vi "Dio3232.vi"(7 "DIO3232_Action":T2, 8 "error in (no error)":errorcluster, 11 "I/Oin":T1 {"Port" items=["input_port0", "input_port1", "input_port2", "input_port3", "output_port0", "output_port1", "output_port2", "output_port3"]; "Point" max=31}) -> (0 "error out":errorcluster, 3 "I/O out":T1 {"Port" items=["input_port0", "input_port1", "input_port2", "input_port3", "output_port0", "output_port1", "output_port2", "output_port3"]})   [LabVIEW 2015]
uses:
  Dio3232_controls.ctl
panel:
  # "input_port0  ÂI¦ìinput0~7\ninput_port1  ÂI¦ìinput8~15\ninput_port2  ÂI¦ìinput16~23\ninput_port3  ÂI¦ìinput24~31"
  # "output_port0  ÂI¦ìoutput0~7\noutput_port1  ÂI¦ìoutput8~15\noutput_port2  ÂI¦ìoutput16~23\noutput_port3  ÂI¦ìoutput24~31"
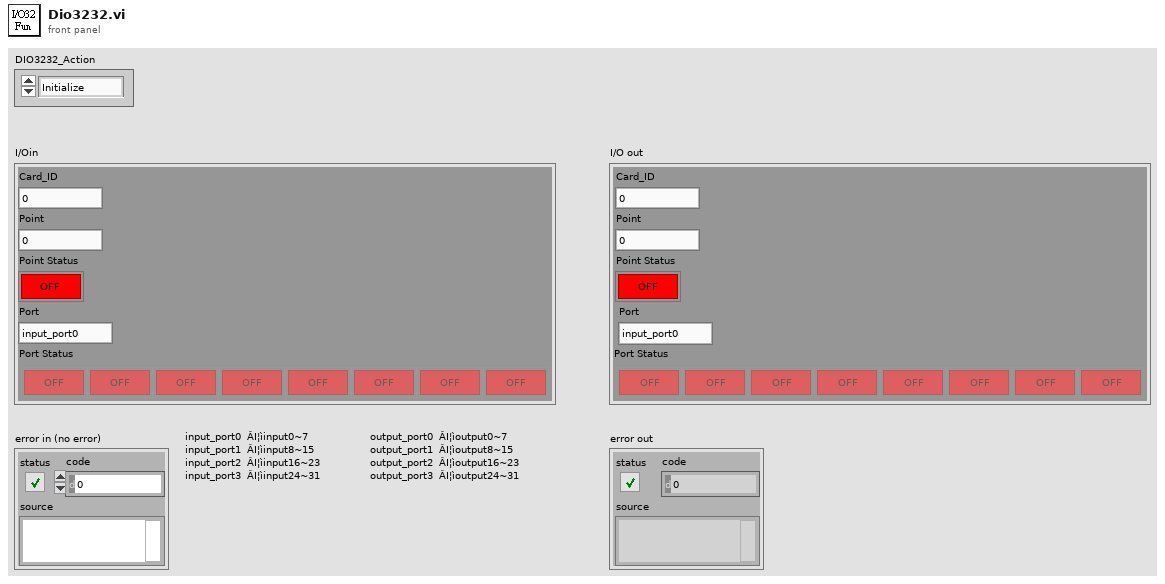
[diagram p1: front panel]
types:
  T1 = cluster{"Card_ID":u8, "Point":u16, "Point Status":bool, "Port":u8, "Port Status":bool[]}
  T2 = typedef "Dio3232_controls.ctl" = enum16{"Initialize", "read_in_point", "read_out_point", "read_port", "set_out_point", "set_port", "close", "Idle"}
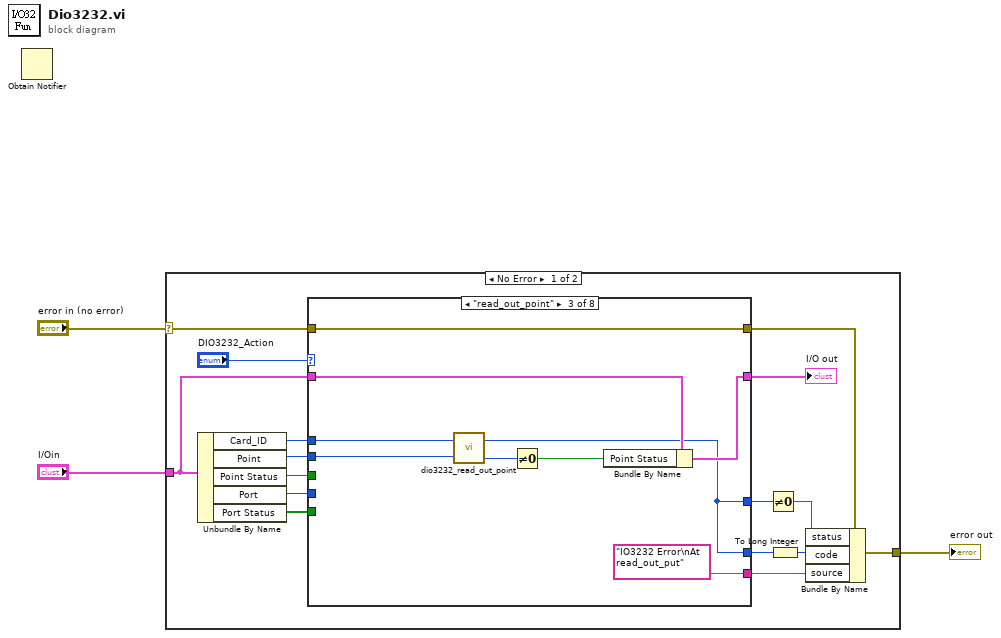
[diagram p0: block diagram]
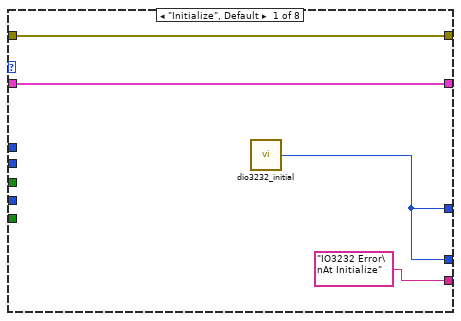
[diagram p2: hidden frame]
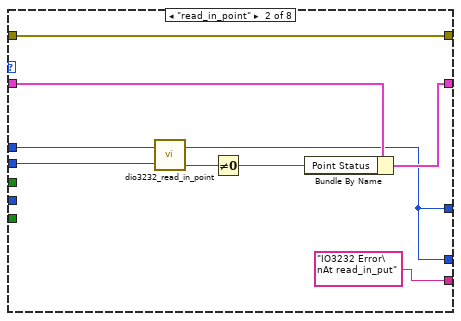
[diagram p3: hidden frame]
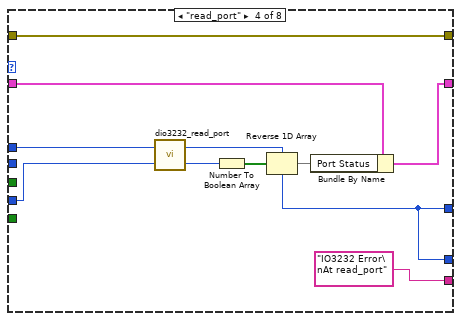
[diagram p4: hidden frame]
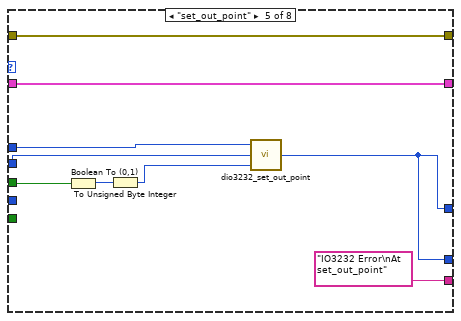
[diagram p5: hidden frame]
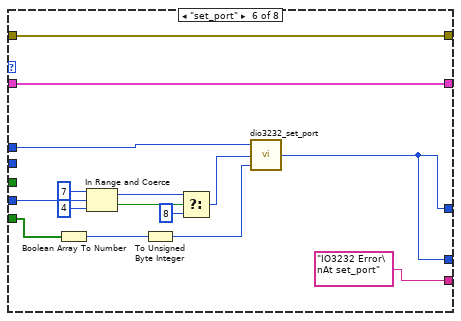
[diagram p6: hidden frame]
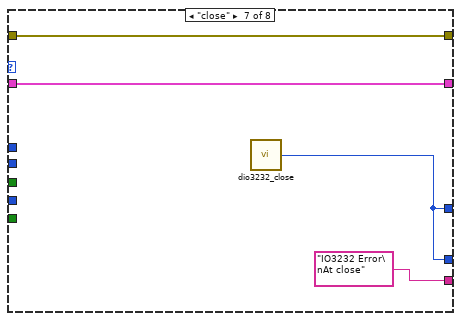
[diagram p7: hidden frame]
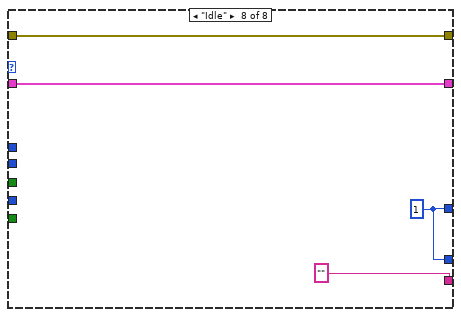
[diagram p8: hidden frame]
diagram:
  n1 = Obtain Notifier() -> ()  [unwired: 4 in, 3 out]
  n2 = case shown="No Error" "error in (no error)" {
    selector: "error in (no error)" -> [w16 w84]
    tunnel: "I/Oin" -> [w18 _]
    tunnel: [w14 w84] -> w1
    frame No Error {
      n3 = Unbundle By Name(w18) -> ("Card_ID"=w13:u8, "Point"=w11:u16, "Point Status"=w7:bool, "Port"=w8:u8, "Port Status"=w6:bool[])
      n4 = case shown="\"read_out_point\"" "DIO3232_Action" {
        tunnel: w18 -> [w23 w29 w37 w48 w53 w74 w78 w82]
        tunnel: [w23 w28 w36 w47 w53 w74 w78 w82] -> w17
        tunnel: w16 -> [w22 w32 w41 w51 w60 w75 w79 w83]
        tunnel: [w22 w32 w41 w51 w60 w75 w79 w83] -> w15
        tunnel: w13 -> [_ w31 w40 w50 w59 w73 _ _]
        tunnel: [w20 w24 w33 w45 w52 w61 w76 w81] -> w10
        tunnel: ["IO3232 Error\nAt Initialize" "IO3232 Error\nAt read_in_put" "IO3232 Error\nAt read_out_put" "IO3232 Error\nAt read_port" "IO3232 Error\nAt set_out_point" "IO3232 Error\nAt set_port" "IO3232 Error\nAt close" ""] -> w12
        tunnel: w11 -> [_ w30 w39 _ w57 _ _ _]
        tunnel: w8 -> [_ _ _ w44 _ w72 _ _]
        tunnel: w7 -> [_ _ _ _ w56 _ _ _]
        tunnel: w6 -> [_ _ _ _ _ w71 _ _]
        tunnel: [w20 w24 w33 w45 w52 w61 w76 w81] -> w4
        frame "Initialize", Default {
          n5 = call <vilib>:"dio3232_initial.vi"() -> ("error_code"=w20:u32)
        }
        frame "read_in_point" {
          n6 = call <vilib>:"dio3232_read_in_point.vi"("Point"=w30, "CardID"=w31) -> ("State"=w27:u8, "error_code"=w24:u32)
          n7 = Not Equal To 0?(x=w27) -> (x != 0?=w26:bool)
          n8 = Bundle By Name(cluster=w29, "Point Status"=w26) -> (w28:T1)
        }
        frame "read_out_point" {
          n9 = call <vilib>:"dio3232_read_out_point.vi"("Point"=w39, "CardID"=w40) -> ("State"=w34:u8, "error_code"=w33:u32)
          n10 = Not Equal To 0?(x=w34) -> (x != 0?=w35:bool)
          n11 = Bundle By Name(cluster=w37, "Point Status"=w35) -> (w36:T1)
        }
        frame "read_port" {
          n12 = call <vilib>:"dio3232_read_port.vi"("Port"=w44, "CardID"=w50) -> ("Data"=w46:u8, "error_code"=w45:u32)
          n13 = Number To Boolean Array(number=w46) -> (Boolean array=w43:bool[])
          n14 = Reverse 1D Array(array=w43) -> (reversed array=w42:bool[])
          n15 = Bundle By Name(cluster=w48, "Port Status"=w42) -> (w47:T1)
        }
        frame "set_out_point" {
          n16 = Boolean To (0,1)(Boolean=w56) -> (0, 1=w55:i16)
          n17 = To Unsigned Byte Integer(number=w55) -> (unsigned 8bit integer=w54:u8)
          n18 = call <vilib>:"dio3232_set_out_point.vi"("State"=w54, "Point"=w57, "CardID"=w59) -> ("error_code"=w52:u32)
        }
        frame "set_port" {
          n19 = Boolean Array To Number(Boolean array=w71) -> (number=w70:u32)
          n20 = In Range and Coerce(upper limit=u8 7, x=w72, lower limit=u8 4) -> (coerced(x)=w63:u8, In Range?=w67:bool)
          n21 = To Unsigned Byte Integer(number=w70) -> (unsigned 8bit integer=w69:u8)
          n22 = Select(t=w63, s=w67, f=u8 8) -> (s? t:f=w62:u8)
          n23 = call <vilib>:"dio3232_set_port.vi"("Data"=w69, "Port"=w62, "CardID"=w73) -> ("error_code"=w61:u32)
        }
        frame "close" {
          n24 = call <vilib>:"dio3232_close.vi"() -> ("error_code"=w76:u32)
        }
        frame "Idle" {
          w81 = u32 1 ("error_code")
        }
      }
      "I/O out" <- w17
      n25 = Not Equal To 0?(x=w10) -> (x != 0?=w9:bool)
      n26 = To Long Integer(number=w4) -> (32bit integer=w5:i32)
      n27 = Bundle By Name(cluster=w15, "status"=w9, "code"=w5, "source"=w12) -> (w14:errorcluster)
    }
    frame Error {
    }
  }
  "error out" <- w1
